vi "Init.vi"(8 "error in (no error)":errorcluster, 10 "Authorization":refnum<class "Authorization.lvclass">) -> (0 "error out":errorcluster, 3 "Async Authorization out":refnum<class "Async Authorization.lvclass">)   [LabVIEW 2020, in "OAuth2.lvlib" / "Async Authorization.lvclass"]
uses:
  Async Authorization.lvclass
  Async Auth State.ctl
  OAuth2.lvlib
  Authorization/Authorization.lvclass
  Async Auth Result.ctl
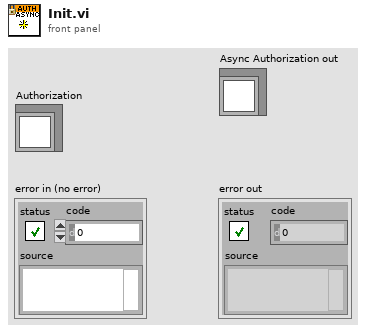
[diagram p1: front panel]
types:
  T1 = typedef "OAuth2.lvlib/Async Auth Result.ctl" = cluster{"Authorization":refnum<class "Authorization.lvclass">, "error":errorcluster}
  T2 = typedef "OAuth2.lvlib/Async Auth State.ctl" = enum16{"Initialize", "Request", "WaitAuth", "GetToken", "RefreshToken", "Complete", "Failed"}
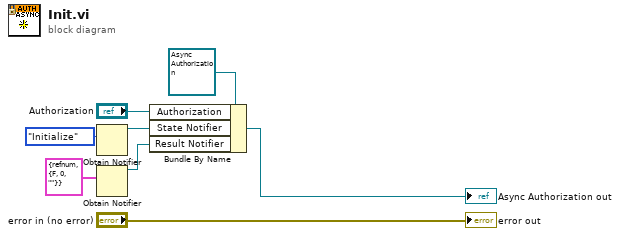
[diagram p0: block diagram]
diagram:
  n1 = Obtain Notifier(notification data type=Async_Auth_State."Initialize" ("Async Auth State")) -> (notifier out=w3:refnum<notifier>)  [unwired: 3 in, 2 out]
  n2 = Obtain Notifier(notification data type=T1 {"Authorization"=refnum, "error"={"status"=FALSE, "code"=0, "source"=""}} ("Result")) -> (notifier out=w1:refnum<notifier>)  [unwired: 3 in, 2 out]
  n3 = Bundle By Name(cluster=refnum<class "Async Authorization.lvclass"> refnum ("Async Authorization in"), "Authorization"="Authorization", "State Notifier"=w3, "Result Notifier"=w1) -> (→"Async Authorization out":refnum<class "Async Authorization.lvclass">)
  "error out" <- "error in (no error)"
